vi "GUNSC_Main.vi"() -> ()   [LabVIEW 2016]
doc: "Main VI for the TCS P60 interface"
uses:
  DBSHAND/private/vis/DatabaseHand_Element_Get(string).vi
  DBSHAND/private/vis/DatabaseHand_Element_Set(I32).vi
  DBSHAND/private/vis/DatabaseHand_Element_Set(string).vi
  DBSHAND/private/vis/DatabaseHand_Element_Get(bool).vi
  DBSHAND/private/vis/DatabaseHand_Element_Set(1DArr).vi
  DBSHAND/private/vis/DatabaseHand_Element_Set(U64).vi
panel:
  in  "libdir":path
  in  "GUNSC command strct":T1
  in  "log":bool
  in  "logfile":path
  in  "key":string
  in  "commands2exec":string
  in  "Extensions":u16[](array[numeric])
  out "num amplifiers":i32
  out "amplifiers":u64
  out "readmode":string
  in  "unscramble struct":T2={"location"=0, "ele Read"=0, "location 2"=0, "bpp"=16}
  out "fits timeout":i32
  out "fitsQueueName":string="unsc2fitsQ"
  in  "OK Button":bool
  in  "local commands":string
  out "error out":errorcluster
  in  "Initialization Variables":string[][](table)=[["MISC", "commands", "GUNSC_Main.vi", "commands2exec", "none", "STR"], ["MISC", "libdir", "GUNSC_Main.vi", "libdir", "", "PATH"], ["LOG", "file", "GUNSC_Main.vi", "logfile", "", "PATH"], ["LOG", "log", "GUNSC_Main.vi", "log", "FALSE", "BOOL"]]
  in  "error in":errorcluster
  out "ConfigFile":path=path "/home/ArcVIEW/Modules/TCSP60/config/TCSP60_Default.cfg"
  in  "ModuleName":string="GUNSC"
  out "Command":string
  out "stopped":bool=TRUE
  out "Reply":string
  in  "ShutDown":bool
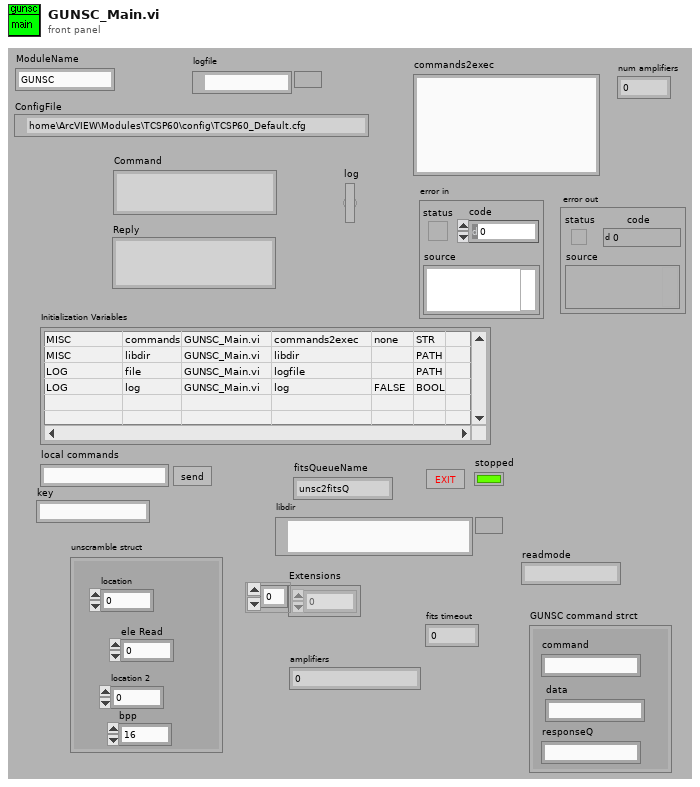
[diagram p1: front panel]
types:
  T1 = cluster{"command":string, "data":string, "responseQ":string}
  T2 = cluster{"location":u64, "ele Read":u32, "location 2":u64, "bpp":i32}
  T3 = cluster{"multiple extensions":bool, "ncols":u16, "nrows":u16, "bpp":i16, "cont_read":bool}
  T4 = typedef "DatabaseHand_RefNum.ctl" = refnum<vi>
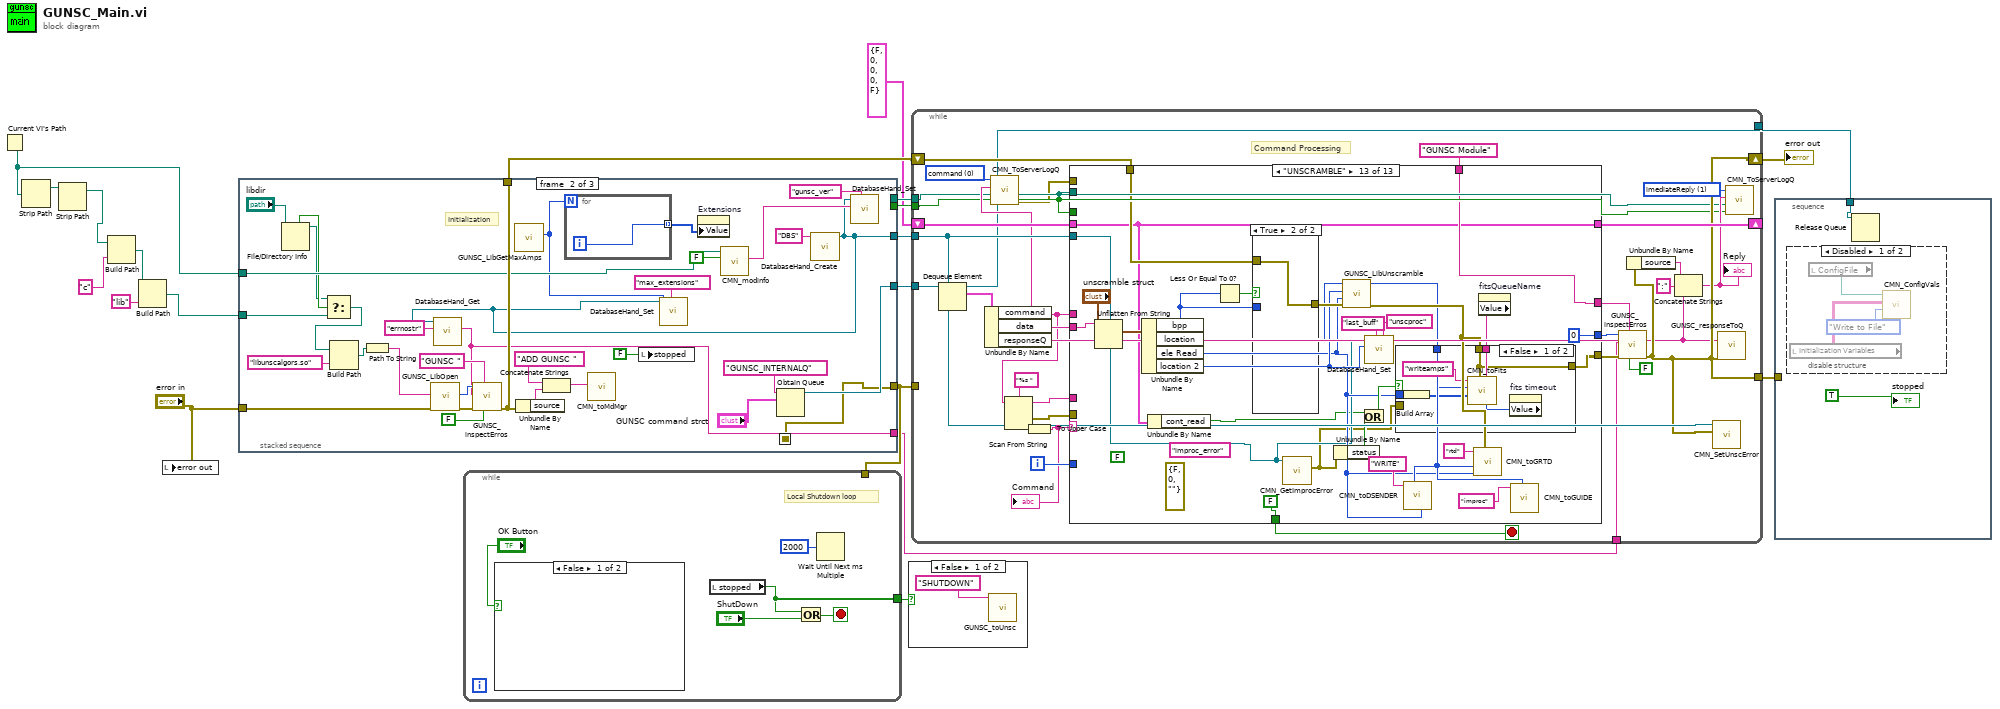
[diagram p0: block diagram]
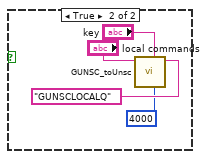
[diagram p3: hidden frame]
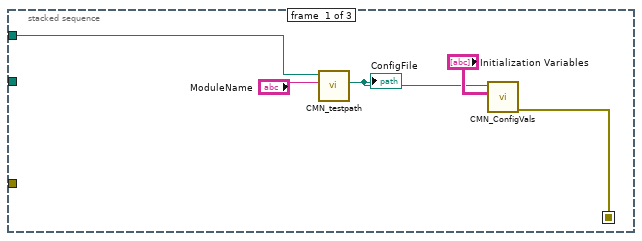
[diagram p5: hidden frame]
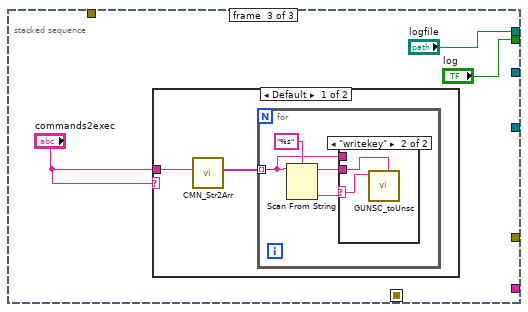
[diagram p6: hidden frame]
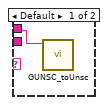
[diagram p7: hidden frame]
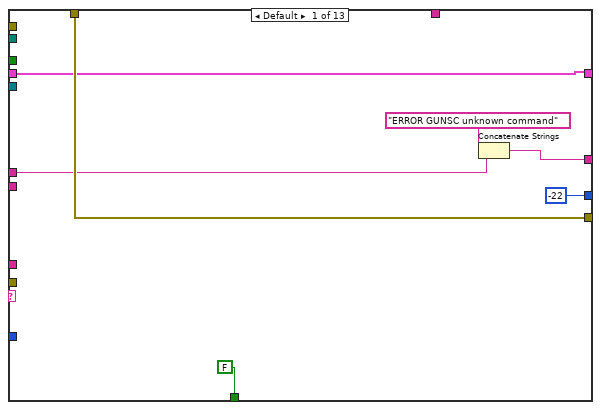
[diagram p9: hidden frame]
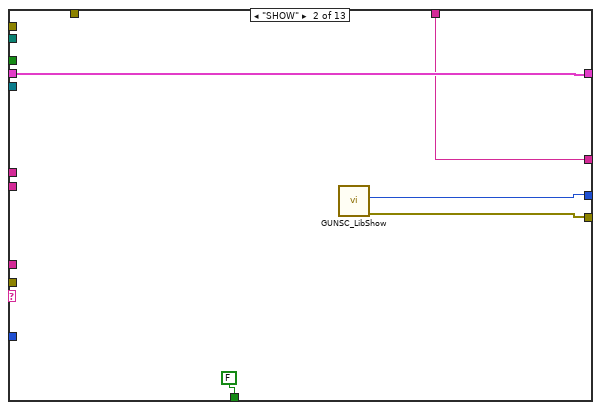
[diagram p10: hidden frame]
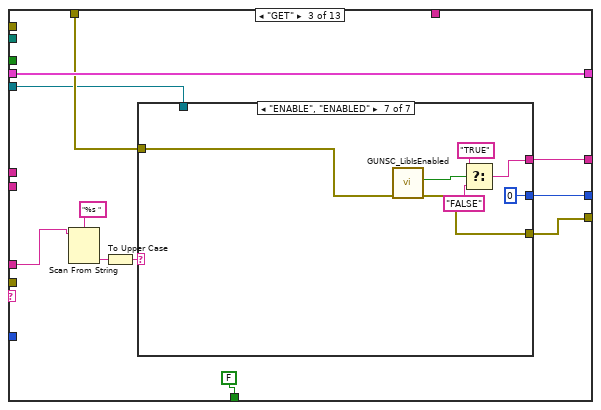
[diagram p11: hidden frame]
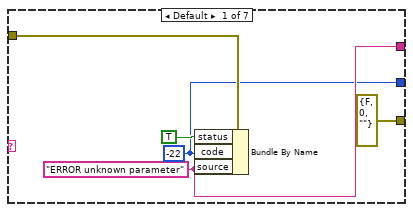
[diagram p12: hidden frame]
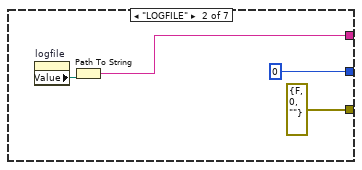
[diagram p13: hidden frame]
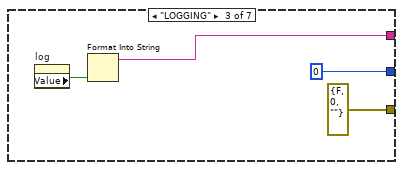
[diagram p14: hidden frame]
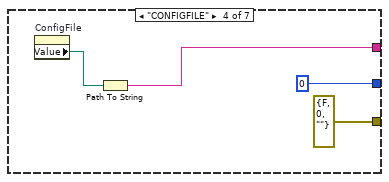
[diagram p15: hidden frame]
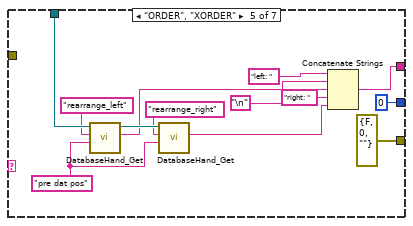
[diagram p16: hidden frame]
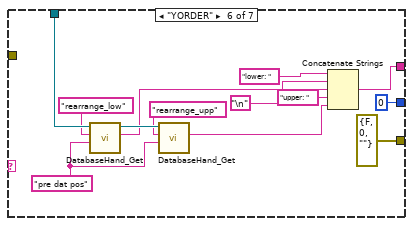
[diagram p17: hidden frame]
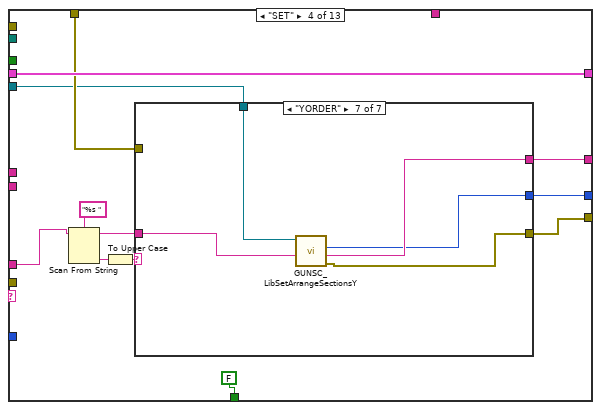
[diagram p18: hidden frame]
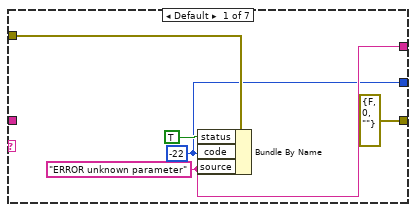
[diagram p19: hidden frame]
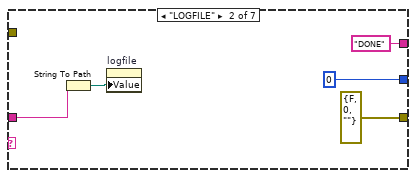
[diagram p20: hidden frame]
diagram:
  n1 = Current VI's Path() -> (path=w1:path)
  n2 = Strip Path(path=w1) -> (stripped path=w11:path)  [unwired: 1 out]
  n3 = Strip Path(path=w11) -> (stripped path=w7:path)  [unwired: 1 out]
  n4 = Build Path(base path=w7, name or relative path="c") -> (appended path=w9:path)
  n5 = Build Path(base path=w9, name or relative path="lib") -> (appended path=w2:path)
  n6 = local write "error out"("error in") -> ()
  n7 = stacked-sequence {
    seq-local: [w21 _ _] -> [_ w36 _]
    tunnel: [_ w36 _] -> w19
    tunnel: "error in" -> [_ w51 _]
    tunnel: [_ w50 _] -> w17
    tunnel: [_ w28 _] -> w14
    tunnel: [_ _ "logfile"] -> w13
    tunnel: [_ _ "log"] -> w12
    tunnel: [_ w41 _] -> w6
    tunnel: [_ w38 _] -> w4
    tunnel: w1 -> [w22 w37 _]
    tunnel: w2 -> [_ w29 _]
    frame #0 {
      n8 = call "CMN_testpath.vi"("ModuleName"="ModuleName", "caller Path"=w22) -> ("ConfigFile"=w24:path)  [unwired: 1 in, 8 out]
      "ConfigFile" <- w24
      n9 = call "CMN_ConfigVals.vi"("ConfigVariables"="Initialization Variables", "configuration file path"=w24) -> ("error out"=w21:errorcluster)  [unwired: 2 in, 7 out]
    }
    frame #1 {
      # "Initialization"
      n10 = File/Directory Info(path="libdir") -> (path out=w33:path, directory=w34:bool)  [unwired: 1 in, 5 out]
      n11 = Select(t=w33, s=w34, f=w29) -> (s? t:f=w30:path)
      n12 = Build Path(base path=w30, name or relative path="libunscalgors.so") -> (appended path=w31:path)
      n13 = Path To String(path=w31) -> (string=w46:string)
      n14 = call "GUNSC_LibOpen.vi"("error in (no error)"=w51, "libpath"=w46) -> ("error out"=w57:errorcluster, "return value"=w56:i32)  [unwired: 8 out]
      n15 = call "GUNSC_LibGetMaxAmps.vi"() -> ("max amps"=w27:i32)  [unwired: 1 in, 10 out]
      n16 = for {
        N: w27 -> [_]
        tunnel: [w59] -> w49 mode=indexing
        i -> [w59]
      }
      n17 = local write "stopped"(FALSE ("stopped")) -> ()
      n18 = property on="Extensions" class="Arr (strict)"("Value"=w49) -> ()  [unwired: 2 in, 2 out]
      n19 = call "CMN_modinfo.vi"("full"=FALSE, "caller path"=w37) -> ("INFO"=w43:string)  [unwired: 1 in, 8 out]
      n20 = Obtain Queue(name (unnamed)="GUNSC_INTERNALQ", element data type="GUNSC command strct") -> (queue out=w38:refnum<queue>)  [unwired: 3 in, 2 out]
      n21 = call "DatabaseHand_Create.vi"("Name"="DBS") -> ("Database RefNum out"=w28:T4)  [unwired: 1 in, 9 out]
      n22 = call-poly "DatabaseHand_Get.vi"("name"="errnostr", "Database RefNum in"=w28) -> ("value"=w41:string)  [unwired: 3 in, 6 out]
      n23 = call "GUNSC_inspectErros.vi"("show Dialog?"=FALSE, "message"="GUNSC ", "error in (no error)"=w57, "errostr"=w41, "error code"=w56) -> ("error out"=w50:errorcluster)  [unwired: 6 out]
      n24 = Unbundle By Name(w50) -> ("source"=w54:string)
      n25 = Concatenate Strings("ADD GUNSC " ("command"), w54) -> (w52:string)
      n26 = call "CMN_toMdMgr.vi"("command"=w52) -> ()  [unwired: 10 out]
      n27 = call-poly "DatabaseHand_Set.vi"("name"="max_extensions", "value"=w27, "Database RefNum in"=w28) -> ()  [unwired: 5 in, 4 out]
      n28 = call-poly "DatabaseHand_Set.vi"("name"="gunsc_ver", "value"=w43, "Database RefNum in"=w28) -> ()  [unwired: 5 in, 4 out]
    }
    frame #2 {
      n29 = case shown="Default" "commands2exec" {
        tunnel: "commands2exec" -> [w64 _]
        frame Default {
          n30 = call "CMN_Str2Arr.vi"("string in"=w64) -> ("Array out"=w63:string[])  [unwired: 3 in, 7 out]
          n31 = for {
            tunnel: w63 -> [w66] mode=indexing
            n32 = Scan From String(format string="%s", input string=w66) -> (remaining string=w65:string, output 1=w67:string)  [unwired: 2 in, 3 out]
            n33 = case shown="\"writekey\"" w67 {
              selector: w67 -> [_ w71]
              tunnel: w66 -> [w69 _]
              tunnel: w65 -> [_ w70]
              frame Default {
                n34 = call "GUNSC_toUnsc.vi"("command"=w69) -> ()  [unwired: 8 in, 3 out]
              }
              frame "writekey" {
                n35 = call "GUNSC_toUnsc.vi"("key"=w70, "command"=w71) -> ()  [unwired: 7 in, 3 out]
              }
            }
          }
        }
        frame "", " ", "none" {
        }
      }
    }
  }
  n36 = while {
    tunnel: [w74] -> w20
    tunnel: w19 -> [_]
    stop <- w76 stop-if-true
    # "Local Shutdown loop"
    n37 = case shown="False" "OK Button" {
      frame False {
      }
      frame True {
        n38 = call "GUNSC_toUnsc.vi"("responseQ"="GUNSCLOCALQ", "ms timeout (-1)"=4000, "key"="key", "command"="local commands") -> ()  [unwired: 5 in, 3 out]
      }
    }
    n39 = local read "stopped"() -> (w74:bool)
    n40 = Or(x=w74, y="ShutDown") -> (x .or. y?=w76:bool)
    n41 = Wait Until Next ms Multiple(millisecond multiple=u32 2000) -> ()  [unwired: 1 out]
  }
  n42 = case shown="False" w20 {
    frame False {
      n43 = call "GUNSC_toUnsc.vi"("command"="SHUTDOWN" ("Command")) -> ()  [unwired: 8 in, 3 out]
    }
    frame True {
    }
  }
  n44 = while {
    tunnel: w19 -> [_]
    shift-right: [w96] -> w18
    shift-left: w17 -> [w105]
    shift-right: [w99] -> _
    shift-left: T3 {"multiple extensions"=FALSE, "ncols"=0, "nrows"=0, "bpp"=0, "cont_read"=FALSE} ("image struct") -> [w98]
    tunnel: [w96] -> w15
    tunnel: w14 -> [w97]
    tunnel: w13 -> [w88]
    tunnel: w12 -> [w87]
    tunnel: w6 -> [w85]
    tunnel: w4 -> [w84]
    tunnel: [w82] -> w3
    i -> [w112]
    stop <- w113 stop-if-true
    w90 = u16 0 items=["command", "imediateReply", "Callback Reply", "Information"] ("type")
    w91 = u16 1 items=["command", "imediateReply", "Callback Reply", "Information"] ("type")
    # "Command Processing"
    n45 = Dequeue Element(queue=w84) -> (queue out=w82:refnum<queue>, element=w83:T1)  [unwired: 1 in, 3 out]
    n46 = Unbundle By Name(w83) -> ("command"=w89:string, "data"=w103:string, "responseQ"=w93:string)
    n47 = call "CMN_ToServerLogQ.vi"("Log"=w87, "file"=w88, "string"=w89, "type"=w90) -> ("error out"=w86:errorcluster)  [unwired: 2 in, 4 out]
    n48 = Scan From String(format string="%s ", input string=w89) -> (remaining string=w108:string, error out=w110:errorcluster, output 1=w109:string)  [unwired: 2 in, 2 out]
    n49 = To Upper Case(1:w109) -> (0:w107:string)
    "Command" <- w107
    n50 = case shown="\"UNSCRAMBLE\"" w107 {
      tunnel: [FALSE FALSE FALSE FALSE FALSE FALSE TRUE FALSE FALSE FALSE FALSE FALSE FALSE] -> w113
      tunnel: w110 -> [_ _ _ _ _ _ _ _ _ _ _ _ _]
      tunnel: w112 -> [_ _ _ _ _ _ _ _ _ _ _ _ _]
      tunnel: w108 -> [_ _ w133 w195 w259 _ _ _ _ _ _ _ _]
      tunnel: w105 -> [w118 _ w127 w189 w256 _ _ w326 _ _ _ _ w471]
      tunnel: [w118 w124 w128 w190 errorcluster {"status"=FALSE, "code"=0, "source"=""} ("error out") w282 w312 w326 w337 w424 w454 w457 w463] -> w104
      tunnel: w103 -> [_ _ _ _ _ _ _ _ w334 _ w452 _ w490]
      tunnel: [-22 w123 w130 w192 w253 0 ("return value") w311 0 w329 w434 w453 w456 0 ("return value")] -> w102
      tunnel: w89 -> [w116 _ _ _ _ _ _ _ _ _ _ _ _]
      tunnel: "GUNSC Module" ("message") -> [_ w122 _ _ _ w308 w314 w321 _ w437 w445 _ w483]
      tunnel: [w115 w122 w129 w191 w251 w308 w314 w319 w330 w437 w445 w458 w483] -> w100
      tunnel: [w114 w125 w136 w198 w262 w310 w313 w318 w338 w435 w446 w462 w470] -> w99
      tunnel: w98 -> [w114 w125 w136 w198 w262 w310 w313 w318 w339 _ w446 w462 w470]
      tunnel: w97 -> [_ _ w126 w187 _ w281 _ _ w336 w431 _ _ w466]
      tunnel: w88 -> [_ _ _ _ _ _ _ _ w333 _ _ _ _]
      tunnel: w87 -> [_ _ _ _ _ _ _ _ w332 _ _ _ _]
      tunnel: w86 -> [_ _ _ _ _ _ _ _ w331 _ _ _ _]
      frame Default {
        n51 = Concatenate Strings("ERROR GUNSC unknown command", w116) -> (w115:string)
      }
      frame "SHOW" {
        n52 = call "GUNSC_LibShow.vi"() -> ("error out"=w124:errorcluster, "return value"=w123:i32)  [unwired: 1 in, 9 out]
      }
      frame "GET" {
        n53 = Scan From String(format string="%s ", input string=w133) -> (output 1=w132:string)  [unwired: 2 in, 4 out]
        n54 = To Upper Case(1:w132) -> (0:w131:string)
        n55 = case shown="\"ENABLE\", \"ENABLED\"" w131 {
          tunnel: [w138 0 ("return value") 0 ("return value") 0 ("return value") 0 ("return value") 0 ("return value") 0 ("return value")] -> w130
          tunnel: [w139 w143 w146 w152 w156 w169 w180] -> w129
          tunnel: [errorcluster {"status"=FALSE, "code"=0, "source"=""} ("error out") errorcluster {"status"=FALSE, "code"=0, "source"=""} ("error out") errorcluster {"status"=FALSE, "code"=0, "source"=""} ("error out") errorcluster {"status"=FALSE, "code"=0, "source"=""} ("error out") errorcluster {"status"=FALSE, "code"=0, "source"=""} ("error out") errorcluster {"status"=FALSE, "code"=0, "source"=""} ("error out") w185] -> w128
          tunnel: w127 -> [w141 _ _ _ _ _ w186]
          tunnel: w126 -> [_ _ _ _ w166 w179 _]
          frame Default {
            w139 = "ERROR unknown parameter" ("source")
            w138 = -22 ("code")
            n56 = Bundle By Name(cluster=w141, "status"=TRUE, "code"=w138, "source"=w139) -> ()  [unwired: 1 out]
          }
          frame "LOGFILE" {
            n57 = property on="logfile" class="Path"() -> ("Value"=w144:path)  [unwired: 2 in, 2 out]
            n58 = Path To String(path=w144) -> (string=w143:string)
          }
          frame "LOGGING" {
            n59 = property on="log" class="Bool (strict)"() -> ("Value"=w147:bool)  [unwired: 2 in, 2 out]
            n60 = Format Into String(w147) -> (resulting string=w146:string)  [unwired: 3 in, 1 out]
          }
          frame "CONFIGFILE" {
            n61 = property on="ConfigFile" class="Path"() -> ("Value"=w150:path)  [unwired: 2 in, 2 out]
            n62 = Path To String(path=w150) -> (string=w152:string)
          }
          frame "ORDER", "XORDER" {
            w162 = "pre dat pos" ("default value")
            n63 = call-poly "DatabaseHand_Get.vi"("default value"=w162, "name"="rearrange_left", "Database RefNum in"=w166) -> ("value"=w160:string, "Database RefNum out"=w164:T4)  [unwired: 2 in, 5 out]
            n64 = call-poly "DatabaseHand_Get.vi"("default value"=w162, "name"="rearrange_right", "Database RefNum in"=w164) -> ("value"=w157:string)  [unwired: 2 in, 6 out]
            n65 = Concatenate Strings("left: " ("string"), w160, "\n", "right: " ("string"), w157) -> (w156:string)
          }
          frame "YORDER" {
            w175 = "pre dat pos" ("default value")
            n66 = call-poly "DatabaseHand_Get.vi"("default value"=w175, "name"="rearrange_low", "Database RefNum in"=w179) -> ("value"=w173:string, "Database RefNum out"=w177:T4)  [unwired: 2 in, 5 out]
            n67 = call-poly "DatabaseHand_Get.vi"("default value"=w175, "name"="rearrange_upp", "Database RefNum in"=w177) -> ("value"=w170:string)  [unwired: 2 in, 6 out]
            n68 = Concatenate Strings("lower: " ("string"), w173, "\n", "upper: " ("string"), w170) -> (w169:string)
          }
          frame "ENABLE", "ENABLED" {
            n69 = call "GUNSC_LibIsEnabled.vi"("error in (no error)"=w186) -> ("error out"=w185:errorcluster, "enabled"=w183:bool)  [unwired: 9 out]
            n70 = Select(t="TRUE", s=w183, f="FALSE") -> (s? t:f=w180:string)
          }
        }
      }
      frame "SET" {
        n71 = Scan From String(format string="%s ", input string=w195) -> (remaining string=w188:string, output 1=w194:string)  [unwired: 2 in, 3 out]
        n72 = To Upper Case(1:w194) -> (0:w193:string)
        n73 = case shown="\"YORDER\"" w193 {
          tunnel: [w200 0 ("return value") w210 -1 ("return value") 0 ("return value") w242 w247] -> w192
          tunnel: [w201 "DONE" ("source") w211 "ERROR read-only" ("source") "DONE" ("source") w243 w248] -> w191
          tunnel: [errorcluster {"status"=FALSE, "code"=0, "source"=""} ("error out") errorcluster {"status"=FALSE, "code"=0, "source"=""} ("error out") w209 errorcluster {"status"=FALSE, "code"=0, "source"=""} ("error out") w232 w244 w249] -> w190
          tunnel: w189 -> [w203 _ _ _ _ _ _]
          tunnel: w188 -> [_ w206 w215 _ w237 w241 w246]
          tunnel: w187 -> [_ _ _ _ _ w240 w245]
          frame Default {
            w201 = "ERROR unknown parameter" ("source")
            w200 = -22 ("code")
            n74 = Bundle By Name(cluster=w203, "status"=TRUE, "code"=w200, "source"=w201) -> ()  [unwired: 1 out]
          }
          frame "LOGFILE" {
            n75 = String To Path(string=w206) -> (path=w205:path)
            n76 = property on="logfile" class="Path"("Value"=w205) -> ()  [unwired: 2 in, 2 out]
          }
          frame "LOGGING" {
            n77 = Scan From String(format string="%s", input string=w215) -> (output 1=w213:string)  [unwired: 2 in, 4 out]
            n78 = To Lower Case(string=w213) -> (all lower case string=w212:string)
            n79 = case shown="Default" w212 {
              tunnel: ["ERROR <on | off>" ("source") "DONE" ("source") "DONE" ("source")] -> w211
              tunnel: [-22 ("return value") 0 ("return value") 0 ("return value")] -> w210
              tunnel: [errorcluster {"status"=FALSE, "code"=0, "source"=""} ("error out") errorcluster {"status"=FALSE, "code"=0, "source"=""} ("error out") errorcluster {"status"=FALSE, "code"=0, "source"=""} ("error out")] -> w209
              frame Default {
              }
              frame "on", "true", "yes" {
                n80 = property on="log" class="Bool (strict)"("Value"=TRUE ("log")) -> ()  [unwired: 2 in, 2 out]
              }
              frame "false", "no", "off" {
                n81 = property on="log" class="Bool (strict)"("Value"=FALSE ("log")) -> ()  [unwired: 2 in, 2 out]
              }
            }
          }
          frame "CONFIGFILE" {
          }
          frame "PIX_SWAP" {
            n82 = Scan From String(format string="%d", input string=w237) -> (error out=w235:errorcluster, output 1=w234:i32)  [unwired: 2 in, 3 out]
            n83 = case shown="Error" w235 {
              tunnel: w234 -> [w238 _]
              tunnel: [w238 0] -> w233
              frame No Error {
              }
              frame Error {
              }
            }
            n84 = call "GUNSC_LibSetSwapPix.vi"("flag"=w233) -> ("error out"=w232:errorcluster)  [unwired: 1 in, 9 out]
          }
          frame "ORDER", "XORDER" {
            n85 = call "GUNSC_LibSetArrangeSections.vi"("how"=w241, "Database RefNum out"=w240) -> ("error out"=w244:errorcluster, "response"=w243:string, "return value"=w242:i32)  [unwired: 1 in, 6 out]
          }
          frame "YORDER" {
            n86 = call "GUNSC_LibSetArrangeSectionsY.vi"("how"=w246, "Database RefNum out"=w245) -> ("error out"=w249:errorcluster, "response"=w248:string, "return value"=w247:i32)  [unwired: 1 in, 6 out]
          }
        }
      }
      frame "ENABLE" {
        n87 = Scan From String(format string="%s ", input string=w259) -> (remaining string=w255:string, output 1=w258:string)  [unwired: 2 in, 3 out]
        n88 = To Upper Case(1:w258) -> (0:w257:string)
        n89 = case shown="Default" w257 {
          tunnel: [errorcluster {"status"=TRUE, "code"=0, "source"=""} ("error out") errorcluster {"status"=FALSE, "code"=0, "source"=""} ("error out") errorcluster {"status"=FALSE, "code"=0, "source"=""} ("error out")] -> w254
          tunnel: w256 -> [_ _ _]
          tunnel: w255 -> [_ _ _]
          tunnel: [FALSE ("flag") TRUE ("flag") FALSE ("flag")] -> w252
          frame Default {
          }
          frame "1", "ON", "TRUE", "YES" {
          }
          frame "0", "FALSE", "NO", "OFF" {
          }
        }
        n90 = case shown="Error" w254 {
          tunnel: [w265 0 ("return value")] -> w253
          tunnel: w252 -> [w264 _]
          tunnel: ["DONE" ("source") w267] -> w251
          frame No Error {
            n91 = call "GUNSC_LibEnable.vi"("flag"=w264) -> ("return value"=w265:i32)  [unwired: 1 in, 9 out]
          }
          frame Error {
            n92 = call "GUNSC_LibIsEnabled.vi"() -> ("enabled"=w270:bool)  [unwired: 1 in, 10 out]
            n93 = Select(t="TRUE", s=w270, f="FALSE") -> (s? t:f=w267:string)
          }
        }
      }
      frame "INIT" {
        w290 = 6000 ("ms timeout (-1)")
        w286 = "UNSCINITQ" ("response Q")
        n94 = call-poly "DatabaseHand_Get.vi"("default value"=FALSE, "name"="detext", "Database RefNum in"=w281) -> ("value"=w278:bool)  [unwired: 2 in, 6 out]
        n95 = call "GUNSC_LibClearAmps.vi"() -> ("error out"=w307:errorcluster)  [unwired: 1 in, 10 out]
        n96 = local read "readmode"() -> (w303:string)
        n97 = call "GUNSC_LibGetFPA.vi"("Extensions"="Extensions", "error in (no error)"=w307, "readmode"=w303, "detext"=w278) -> ("error out"=w305:errorcluster, "num amplifiers"=w300:i32, "Extensions_out"=w288:u16[], "totysize"=w292:i32, "totxsize"=w293:i32)  [unwired: 3 out]
        "num amplifiers" <- w300
        n98 = local write "Extensions"(w288) -> ()
        n99 = Format Into String(format string="num_amplifiers %d" ("string"), w300) -> (resulting string=w299:string)  [unwired: 2 in, 1 out]
        n100 = Format Into String(format string="totsize %d %d", w293, w292) -> (resulting string=w294:string)  [unwired: 2 in, 1 out]
        n101 = call "GUNSC_LibGetAmpsPtr.vi"("error in (no error)"=w305) -> ("error out"=w289:errorcluster, "return value"=w277:u64)  [unwired: 9 out]
        "amplifiers" <- w277
        n102 = call "CMN_toFits.vi"("ms timeout (-1)"=w290, "response Q"=w286, "key"=w299, "error in (no error)"=w289, "command"="writekey") -> ("error out"=w298:errorcluster)  [unwired: 3 in, 3 out]
        n103 = call "CMN_toGRTD.vi"("location"=w277, "Command"="INIT") -> ()  [unwired: 6 in, 4 out]
        n104 = call "CMN_toFits.vi"("ms timeout (-1)"=w290, "response Q"=w286, "key"=w294, "error in (no error)"=w298, "command"="writekey") -> ("error out"=w297:errorcluster)  [unwired: 3 in, 3 out]
        n105 = call "CMN_toFits.vi"("ms timeout (-1)"=w290, "error in (no error)"=w297, "location"=w277, "command"="INIT") -> ("error out"=w285:errorcluster)  [unwired: 4 in, 3 out]
        n106 = call "CMN_toGUIDE.vi"("pointer"=w277, "error in (no error)"=w285, "Command"="INIT") -> ("error out"=w282:errorcluster)  [unwired: 2 in, 6 out]
        n107 = call "CMN_toDSENDER.vi"("pointer"=w277, "error in (no error)"=w282, "Command"="INIT") -> ()  [unwired: 4 in, 5 out]
      }
      frame "SHUTDOWN" {
        n108 = call "CMN_toMdMgr.vi"("command"="DELETE GUNSC shutdown" ("element")) -> ()  [unwired: 10 out]
        n109 = local write "stopped"(TRUE ("stopped")) -> ()
        n110 = call "GUNSC_LibClose.vi"() -> ("error out"=w312:errorcluster, "return value"=w311:i32)  [unwired: 1 in, 9 out]
      }
      frame "STATE" {
        n111 = Unbundle By Name(w326) -> ("source"=w324:string)
        n112 = Concatenate Strings("ERROR ", w324) -> (w323:string)
        n113 = Select(t=w323, s=w326, f="OK") -> (s? t:f=w320:string)
        n114 = Concatenate Strings(w321, w320) -> (w319:string)
      }
      frame "WRITEKEY" {
        w335 = u16 0 items=["command", "imediateReply", "Callback Reply", "Information"] ("type")
        n115 = Scan From String(format string="%s" ("Format String"), input string=w334) -> (remaining string=w340:string, output 1=w341:string)  [unwired: 2 in, 3 out]
        n116 = call "CMN_ToServerLogQ.vi"("error in (no error)"=w331, "Log"=w332, "file"=w333, "string"=w334, "type"=w335) -> ()  [unwired: 1 in, 5 out]
        n117 = case shown="\"get_physmap\"" w341 {
          tunnel: w340 -> [_ w359 w371 w391 w402 w413 _]
          tunnel: w339 -> [w347 w358 w369 w387 w399 w414 w421]
          tunnel: [w347 w357 w369 w387 w399 w414 w421] -> w338
          tunnel: [errorcluster {"status"=TRUE, "code"=-22, "source"="GUNSC unknown command"} ("error IO") w351 errorcluster {"status"=FALSE, "code"=0, "source"=""} ("error IO") w380 w400 w410 errorcluster {"status"=FALSE, "code"=0, "source"=""} ("error out")] -> w337
          tunnel: w336 -> [_ w355 w365 w379 _ w409 w419]
          tunnel: ["ERROR unknown command" ("response") "DONE" ("response") "DONE" ("response") "DONE" ("response") "DONE" ("response") "DONE" ("response") w417] -> w330
          tunnel: [-22 0 0 0 0 w404 0 ("return value")] -> w329
          frame Default {
          }
          frame "bpp" {
            n118 = Decimal String To Number(string=w359) -> (number=w354:i32)  [unwired: 3 out]
            n119 = Bundle By Name(cluster=w358, "bpp"=w354) -> (w357:T3)
            n120 = Format Into String(format string="SET BPP %d", w354) -> (resulting string=w356:string)  [unwired: 2 in, 1 out]
            n121 = call-poly "DatabaseHand_Set.vi"("group"="improc", "name"="bpp", "value"=w354, "Database RefNum in"=w355) -> ("error out"=w351:errorcluster)  [unwired: 4 in, 3 out]
            n122 = call "CMN_toDBS.vi"("command"=w356) -> ()  [unwired: 3 in, 8 out]
          }
          frame "readmode" {
            n123 = Scan From String(format string="%s", input string=w371) -> (output 1=w363:string)  [unwired: 2 in, 4 out]
            "readmode" <- w363
            n124 = call-poly "DatabaseHand_Set.vi"("group"="improc", "name"="currentreadmode", "value"=w363, "Database RefNum in"=w365) -> ()  [unwired: 4 in, 4 out]
            n125 = Format Into String(format string="SET READMODE %s", w363) -> (resulting string=w368:string)  [unwired: 2 in, 1 out]
            n126 = call "CMN_toDBS.vi"("command"=w368) -> ()  [unwired: 3 in, 8 out]
          }
          frame "waitfits" {
            n127 = Scan From String(format string="%s %d" ("Format String"), input string=w391) -> (error out=w380:errorcluster, output 1=w394:string, output 2=w385:i32)  [unwired: 2 in, 4 out]
            n128 = Max & Min(x=w385, y=200) -> (max(x,y)=w382:i32)  [unwired: 1 out]
            n129 = Less Than 0?(x=w385) -> (x < 0?=w384:bool)
            n130 = call-poly "DatabaseHand_Get.vi"("default value"=FALSE, "name"="fits_present", "Database RefNum in"=w379) -> ("value"=w374:bool)  [unwired: 2 in, 6 out]
            n131 = Match True/False String(2:"no" ("false string"), 3:"yes" ("true string"), 4:w394) -> (0:w375:bool)  [unwired: 1 out]
            n132 = Select(t=-1, s=w384, f=w382) -> (s? t:f=→"fits timeout":i32)
            n133 = And(x=w374, y=w375) -> (x .and. y?=w376:bool)
            n134 = Select(t="unscToFitsQ", s=w376, f="") -> (s? t:f=→"fitsQueueName":string)
          }
          frame "num_amplifiers" {
            n135 = Scan From String(format string="%d", input string=w402) -> (error out=w400:errorcluster, output 1=w398:i32)  [unwired: 2 in, 3 out]
            n136 = local write "num amplifiers"(w398) -> ()
          }
          frame "physmap" {
            n137 = local read "num amplifiers"() -> (w411:i32)
            n138 = call "GUNSC_Str2EXtensions.v.vi"("command"=w413, "max amps"=w411) -> ("error IO"=w412:errorcluster, "Extensions"=w405:u16[])  [unwired: 1 in, 7 out]
            n139 = Number To Decimal String(number=w405) -> (decimal integer string=w408:string[])  [unwired: 1 out]
            n140 = call "GUNSC_LibSetPhyMap.vi"("error in (no error)"=w412, "num_elements"=w411, "array"=w405) -> ("error out"=w410:errorcluster, "return value"=w404:i32)  [unwired: 7 out]
            n141 = call-poly "DatabaseHand_Set.vi"("group"="improc", "name"="ampphysmap", "value"=w408, "Database RefNum in"=w409) -> ()  [unwired: 5 in, 3 out]
            n142 = case shown="No Error" w410 {
              tunnel: w405 -> [w415 _]
              frame No Error {
                n143 = property on="Extensions" class="Arr (strict)"("Value"=w415) -> ()  [unwired: 2 in, 2 out]
              }
              frame Error {
              }
            }
          }
          frame "get_physmap" {
            n144 = local read "num amplifiers"() -> (w418:i32)
            n145 = call "GUNSC_GetPhysMap.vi"("Database RefNum in"=w419, "num amps"=w418) -> ("response"=w417:string)  [unwired: 9 out]
          }
        }
      }
      frame "COMPUTE" {
        n146 = call "GUNSC_GetImageGeom.vi"("Database RefNum"=w431) -> ("name"=w428:string, "image struct"=w435:T3)  [unwired: 9 out]
        n147 = call "CMN_SetUnscError.vi"("unsc error"=errorcluster {"status"=FALSE, "code"=0, "source"=""} ("unscrambling error"), "Database RefNum in"=w431) -> ("error out"=w430:errorcluster)  [unwired: 1 in, 8 out]
        n148 = Unbundle By Name(w435) -> ("cont_read"=w426:bool, "bpp"=w433:i16)
        n149 = Concatenate Strings("compute " ("Command"), w428) -> (w427:string)
        n150 = call "GUNSC_LibSetFunction.vi"("error in (no error)"=w430, "datatype"=w433) -> ("error out"=w423:errorcluster, "return value"=w434:i32)  [unwired: 8 out]
        n151 = local read "amplifiers"() -> (w422:u64)
        n152 = case shown="False" w426 {
          tunnel: w423 -> [w442 _]
          tunnel: w422 -> [w441 _]
          tunnel: [w440 errorcluster {"status"=FALSE, "code"=0, "source"=""} ("error out")] -> w424
          frame False {
            n153 = property on="fitsQueueName" class="Str"() -> ("Value"=w438:string)  [unwired: 2 in, 2 out]
            n154 = property on="fits timeout" class="DigNum (strict)"() -> ("Value"=w439:i32)  [unwired: 2 in, 2 out]
            n155 = call "CMN_toFits.vi"("ms timeout (-1)"=w439, "response Q"=w438, "error in (no error)"=w442, "location"=w441, "command"="create") -> ("error out"=w440:errorcluster)  [unwired: 3 in, 3 out]
          }
          frame True {
          }
        }
        n156 = call "CMN_toDSENDER.vi"("pointer"=w422, "error in (no error)"=w423, "Command"="OPEN") -> ()  [unwired: 4 in, 5 out]
        n157 = call "CMN_toGRTD.vi"("location"=w422, "argument"=w427) -> ()  [unwired: 6 in, 4 out]
      }
      frame "COPY_BUFFER" {
        n158 = local read "unscramble struct"() -> (w451:T2)
        n159 = Unflatten From String(type=w451, binary string=w452) -> (value=w450:T2)  [unwired: 1 in, 4 out]
        n160 = Unbundle By Name(w450) -> ("location"=w449:u64, "ele Read"=w448:u32, "location 2"=w447:u64)
        n161 = call "GUNSC_LibCopyImage.vi"("amplifiers"=w447, "totcols"=w448, "bufptr"=w449) -> ("error out"=w454:errorcluster, "return value"=w453:i32)  [unwired: 1 in, 6 out]
      }
      frame "GET_RAW_PTR" {
        n162 = call "GUNSC_LibGetRawPtr.vi"() -> ("error out"=w457:errorcluster, "namps"=w459:i32, "raw image ptr"=w460:u64)  [unwired: 1 in, 8 out]
        n163 = Format Into String(w460, w459) -> (resulting string=w458:string)  [unwired: 3 in, 1 out]
        n164 = Unbundle By Name(w457) -> ("code"=w456:i32)
      }
      frame "UNSCRAMBLE" {
        (unwired) errorcluster {"status"=FALSE, "code"=0, "source"=""} ("picread Error")
        (unwired) FALSE
        (unwired) "improc_error" ("name")
        n165 = Unflatten From String(type="unscramble struct", binary string=w490) -> (value=w488:T2)  [unwired: 1 in, 4 out]
        n166 = Unbundle By Name(w488) -> ("bpp"=w486:i32, "location"=w484:u64, "ele Read"=w467:u32, "location 2"=w477:u64)
        n167 = Unbundle By Name(w470) -> ("cont_read"=w465:bool)
        n168 = Less Or Equal To 0?(x=w486) -> (x <= 0?=w487:bool)
        n169 = case shown="True" w487 {
          tunnel: w486 -> [w501 _]
          tunnel: w471 -> [w500 w502]
          tunnel: [w499 w502] -> w485
          frame False {
            n170 = call "GUNSC_LibSetFunction.vi"("error in (no error)"=w500, "datatype"=w501) -> ("error out"=w499:errorcluster)  [unwired: 9 out]
          }
          frame True {
          }
        }
        n171 = call "CMN_GetImprocError.vi"("Database RefNum in"=w466) -> ("improc_error"=w464:errorcluster)  [unwired: 1 in, 9 out]
        n172 = Unbundle By Name(w464) -> ("status"=w473:bool)
        n173 = call "GUNSC_LibUnscramble.vi"("error in (no error)"=w485, "nelems"=w467, "imptr"=w477, "rawptr"=w484) -> ("error out"=w479:errorcluster, "return value"=w468:u64)  [unwired: 6 out]
        n174 = Or(x=w465, y=w473) -> (x .or. y?=w472:bool)
        n175 = call-poly "DatabaseHand_Set.vi"("group"="unscproc", "name"="last_buff", "value"=w477, "Database RefNum in"=w466) -> ()  [unwired: 4 in, 4 out]
        n176 = call "CMN_toDSENDER.vi"("nelems"=w467, "pointer"=w468, "Command"="WRITE") -> ()  [unwired: 4 in, 5 out]
        n177 = call "CMN_toGRTD.vi"("error in (no error)"=w479, "Elements Read"=w467, "location"=w468, "Command"="rtd") -> ()  [unwired: 4 in, 4 out]
        n178 = property on="fitsQueueName" class="Str"() -> ("Value"=w480:string)  [unwired: 2 in, 2 out]
        n179 = case shown="False" w472 {
          tunnel: w480 -> [w495 _]
          tunnel: w479 -> [w491 _]
          tunnel: w467 -> [w494 _]
          tunnel: w468 -> [w493 _]
          tunnel: w464 -> [_ w498]
          tunnel: [w491 w498] -> w463
          frame False {
            n180 = Build Array(w494) -> (w496:u32[])
            n181 = property on="fits timeout" class="DigNum (strict)"() -> ("Value"=w492:i32)  [unwired: 2 in, 2 out]
            n182 = call "CMN_toFits.vi"("ms timeout (-1)"=w492, "response Q"=w495, "error in (no error)"=w491, "eleRead"=w496, "location"=w493, "command"="writeamps") -> ()  [unwired: 2 in, 4 out]
          }
          frame True {
          }
        }
        n183 = call "CMN_toGUIDE.vi"("pointer"=w468, "Command"="improc") -> ()  [unwired: 3 in, 7 out]
      }
    }
    n184 = call "GUNSC_inspectErros.vi"("show Dialog?"=FALSE, "message"=w100, "error in (no error)"=w104, "errostr"=w85, "error code"=w102) -> ("error out"=w96:errorcluster)  [unwired: 6 out]
    n185 = Unbundle By Name(w96) -> ("source"=w95:string)
    n186 = Concatenate Strings(w95, ":" ("string"), w93) -> (w92:string)
    "Reply" <- w92
    n187 = call "CMN_SetUnscError.vi"("unsc error"=w96, "Database RefNum in"=w97) -> ()  [unwired: 1 in, 9 out]
    n188 = call "GUNSC_responseToQ.vi"("error in"=w96, "queue name"=w93) -> ()  [unwired: 10 out]
    n189 = call "CMN_ToServerLogQ.vi"("Log"=w87, "file"=w88, "string"=w92, "type"=w91) -> ()  [unwired: 2 in, 5 out]
  }
  "error out" <- w18
  n190 = stacked-sequence {
    tunnel: w15 -> [_]
    tunnel: w3 -> [w503]
    frame #0 {
      n191 = disable-structure shown="Disabled" {
        frame Disabled {
          n192 = local read "Initialization Variables"() -> (w506:string[][])
          n193 = local read "ConfigFile"() -> (w507:path)
          n194 = call "CMN_ConfigVals.vi"("Action"=enum16{"Read from File", "Write to File"}."Write to File", "ConfigVariables"=w506, "configuration file path"=w507) -> ()  [unwired: 8 in, 1 out]
        }
        frame Enabled {
        }
      }
      n195 = Release Queue(queue=w503) -> ()  [unwired: 1 in, 4 out]
      "stopped" <- TRUE
    }
  }
